vi "Write Auto Range.vi"(8 "error in (no error)":errorcluster, 10 "Auto Range":bool, 11 "34401 in":refnum<class "34401.lvclass">) -> (0 "error out":errorcluster, 3 "34401 out":refnum<class "34401.lvclass">)   [LabVIEW 2018, in "34401.lvlib" / "34401.lvclass"]
uses:
  34401.lvclass
  34401.lvclass/34401.ctl
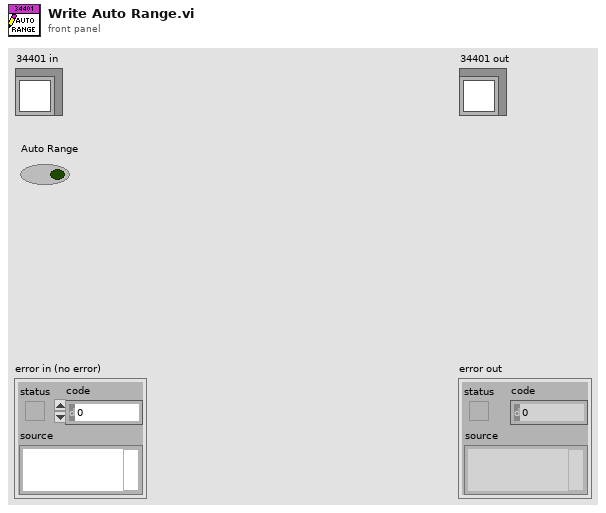
[diagram p1: front panel]
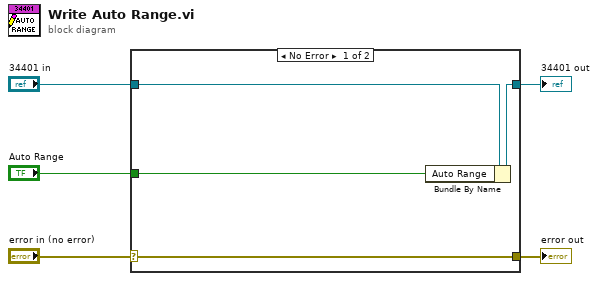
[diagram p0: block diagram]
diagram:
  n1 = case shown="No Error" "error in (no error)" {
    selector: "error in (no error)" -> [w9 w10]
    tunnel: [w9 w10] -> w4
    tunnel: [w7 w11] -> w2
    tunnel: "34401 in" -> [w8 w11]
    tunnel: "Auto Range" -> [w6 _]
    frame No Error {
      n2 = Bundle By Name(cluster=w8, "Auto Range"=w6) -> (w7:refnum<class "34401.lvclass">)
    }
    frame Error {
    }
  }
  "error out" <- w4
  "34401 out" <- w2
